vi "test_CONEX.vi"() -> ()   [LabVIEW 2010]
uses:
  <vilib>/Utility/inputDevices.llb/mouseAcquire.vi
  <vilib>/Utility/inputDevices.llb/closeMouse.vi
panel:
  in  "stop moving":bool
  in  "mouse sensitivity":dbl(slide)=4.94949494949495 scale=0.0..10.0
  in  "move with mouse":bool
  in  "Units":enum16{"mm", "um", "nm"}(ring)=enum."um"
  in  "Goto (incr)":bool
  in  "Motors to move":bool[](array[boolean])=[TRUE, TRUE, TRUE]
  in  "Incr. Stage Move (um)":dbl[](array[numeric])=[0.0, 0.0, 0.0]
  out "moving stage?":bool
  in  "Retract Limit":dbl[](array[numeric])=[0.0, 0.0, 0.0]
  in  "Extend Limit":dbl[](array[numeric])=[12.0, 12.0, 12.0]
  out "Position (mm)":dbl[](array[numeric]) format="%.5g"
  out "CONEX Cluster":T1
  in  "Connected devices":string[](array[string])=["COM3", "COM4", "COM5"]
  in  "Controller Addresses":i32[](array[numeric])=[1, 1, 1]
  in  "Abs. Stage Move":dbl[](array[numeric])=[0.0, 0.0, 0.0]
  in  "Goto (abs)":bool
  in  "stop":bool
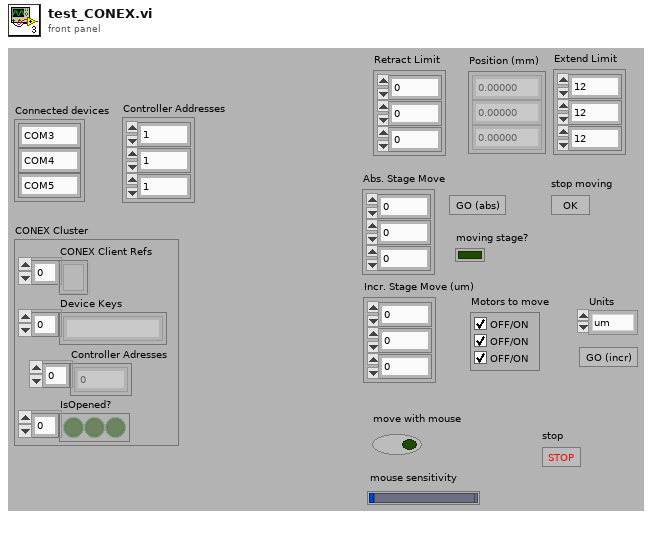
[diagram p1: front panel]
types:
  T1 = cluster{"CONEX Client Refs":refnum<k24>[], "Device Keys":string[], "Controller Adresses":i32[], "IsOpened?":bool[]}
  T2 = cluster{"Horizontal":i32, "Vertical":i32, "Scrolling":i32}
  T3 = cluster{"button 1":bool, "button 2":bool, "button 3":bool, "button 4":bool}
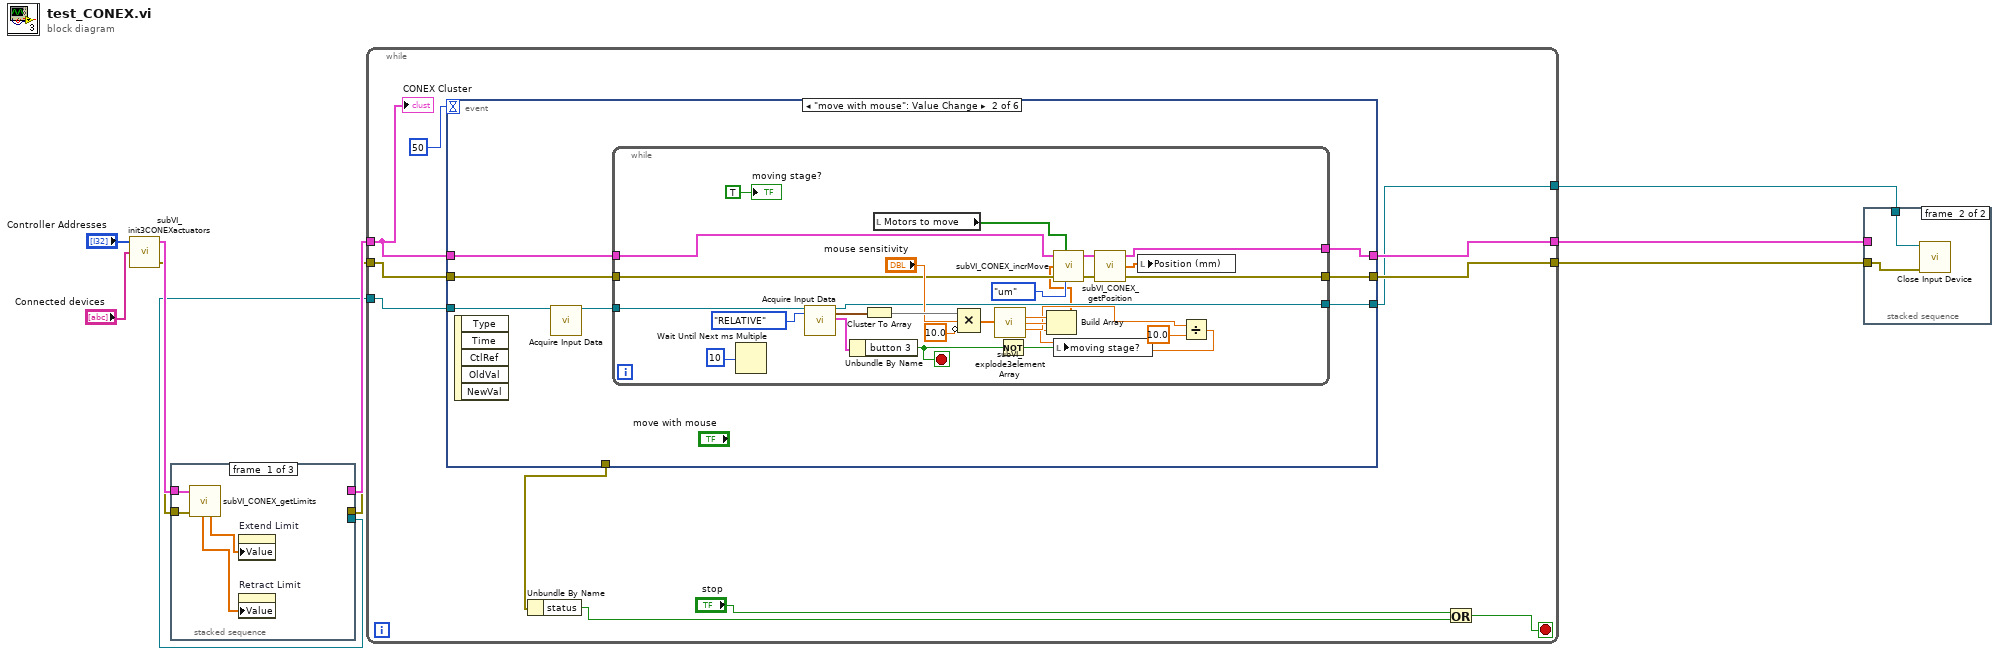
[diagram p0: block diagram]
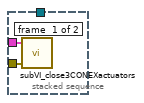
[diagram p2: hidden frame]
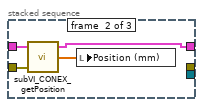
[diagram p3: hidden frame]
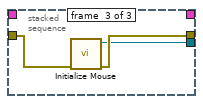
[diagram p4: hidden frame]
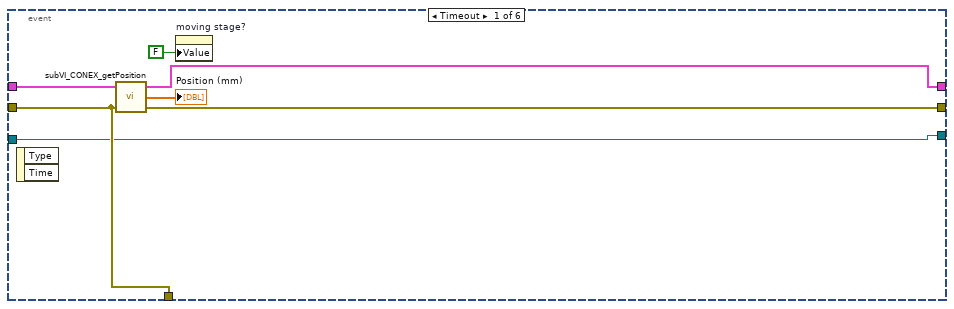
[diagram p5: hidden frame]
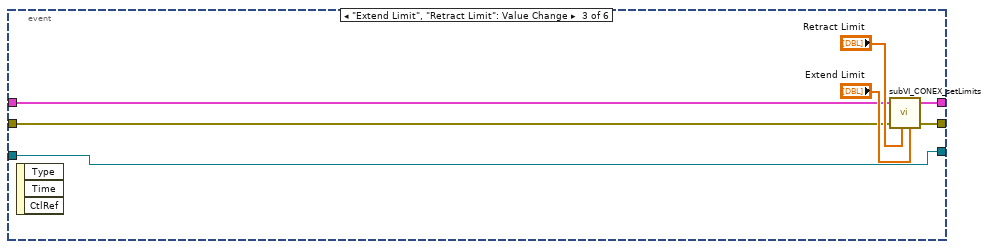
[diagram p6: hidden frame]
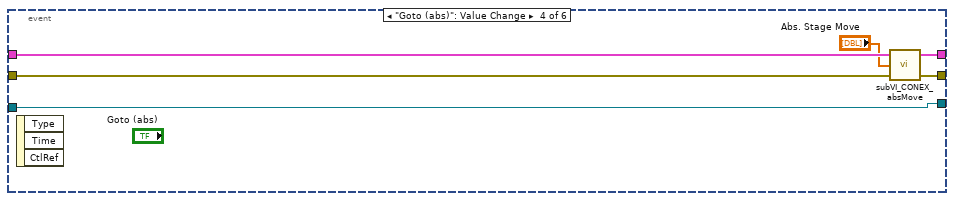
[diagram p7: hidden frame]
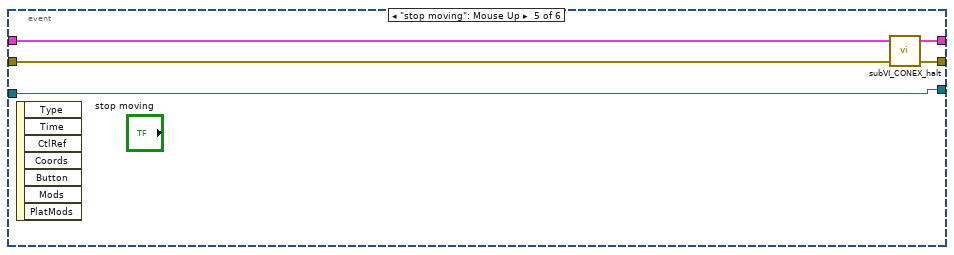
[diagram p8: hidden frame]
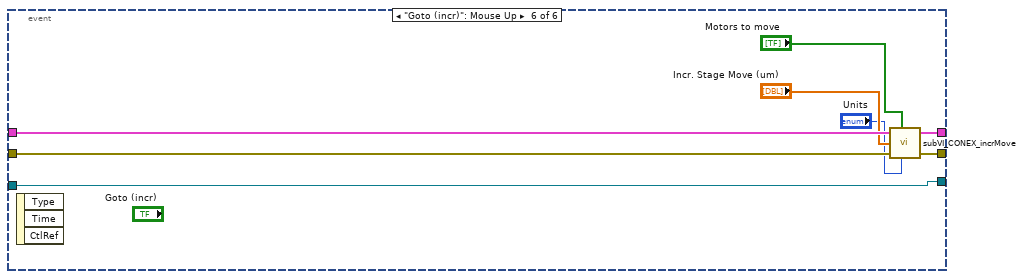
[diagram p9: hidden frame]
diagram:
  n1 = call "subVI_init3CONEXactuators.vi"("Connected devices"="Connected devices", "Controller Addresses"="Controller Addresses") -> ("Error OUT"=w6:errorcluster, "CONEX Cluster"=w7:T1)  [unwired: 2 in]
  n2 = stacked-sequence {
    tunnel: w7 -> [w14 w17 _]
    tunnel: w6 -> [w13 w16 w21]
    tunnel: [_ w15 _] -> w5
    tunnel: [_ _ w20] -> w4
    tunnel: [_ _ w19] -> w2
    frame #0 {
      n3 = call "subVI_CONEX_getLimits.vi"("CONEX Cluster"=w14, "Error IN"=w13) -> ("Retract Limit"=w11:dbl[], "Extend Limit"=w12:dbl[])  [unwired: 4 in, 2 out]
      n4 = property on="Extend Limit" class="Arr (strict)"("Value"=w12) -> ()  [unwired: 2 in, 2 out]
      n5 = property on="Retract Limit" class="Arr (strict)"("Value"=w11) -> ()  [unwired: 2 in, 2 out]
    }
    frame #1 {
      n6 = call "subVI_CONEX_getPosition.vi"("Error IN"=w16, "CONEX Cluster"=w17) -> ("Current Position (mm)"=w18:dbl[], "CONEX Cluster out"=w15:T1)  [unwired: 1 in, 1 out]
      n7 = local write "Position (mm)"(w18) -> ()
    }
    frame #2 {
      n8 = call <vilib>:"Initialize Mouse.vi"("error in (no error)"=w21) -> ("error out"=w20:errorcluster, "device ID"=w19:refnum<k1>)  [unwired: 9 in]
    }
  }
  n9 = while {
    tunnel: w5 -> [w31]
    tunnel: w4 -> [w30]
    tunnel: [w29] -> w10
    tunnel: [w28] -> w3
    tunnel: w2 -> [w23]
    tunnel: [w22] -> w1
    stop <- w24 stop-if-true
    n10 = event shown="[1] \"move with mouse\": Value Change" {
      selector: _ -> [_ _ _ _ _ _]
      dyn-events: _ -> [_ _ _ _ _ _]
      timeout: 50 -> [_ _ _ _ _ _]
      tunnel: w31 -> [w39 w46 w79 w87 w92 w100]
      tunnel: w30 -> [w36 w45 w78 w86 w91 w99]
      tunnel: [w33 w43 w77 w85 w89 w97] -> w29
      tunnel: [w34 w44 w76 w84 w90 w98] -> w28
      tunnel: [w36 _ _ _ _ _] -> w27
      tunnel: w23 -> [w35 w41 w75 w83 w88 w93]
      tunnel: [w35 w42 w75 w83 w88 w93] -> w22
      event Timeout {
        n11 = event-data() -> ()  [unwired: 1 in, 2 out]
        n12 = call "subVI_CONEX_getPosition.vi"("Error IN"=w36, "CONEX Cluster"=w39) -> ("error out"=w33:errorcluster, "Current Position (mm)"=→"Position (mm)":dbl[], "CONEX Cluster out"=w34:T1)  [unwired: 1 in]
        n13 = property on="moving stage?" class="Bool (strict)"("Value"=FALSE ("Boolean")) -> ()  [unwired: 2 in, 2 out]
      }
      event "move with mouse": Value Change {
        n14 = event-data() -> ()  [unwired: 1 in, 5 out]
        n15 = call-poly <vilib>:"Acquire Input Data.vi"("device ID"=w41) -> ("device ID"=w40:refnum<k1>)  [unwired: 15 in, 3 out]
        n16 = while {
          tunnel: w46 -> [w65]
          tunnel: w45 -> [w66]
          tunnel: [w60] -> w44
          tunnel: [w59] -> w43
          tunnel: w40 -> [w74]
          tunnel: [w54] -> w42
          stop <- w55 stop-if-true
          n17 = Wait Until Next ms Multiple(millisecond multiple=u32 10) -> ()  [unwired: 1 out]
          n18 = call-poly <vilib>:"Acquire Input Data.vi"("device ID"=w74, "key mode"=enum16{"RELATIVE", "ABSOLUTE"}."RELATIVE") -> ("device ID"=w54:refnum<k1>, "axis info"=w71:T2, "button info"=w63:T3)  [unwired: 14 in, 1 out]
          n19 = Unbundle By Name(w63) -> ("button 3"=w55:bool)
          n20 = Cluster To Array(cluster=w71) -> (array=w70:i32[])
          n21 = local read "Motors to move"() -> (w64:bool[])
          n22 = Compound Arithmetic op=MULTIPLY(w70, "mouse sensitivity", invert 10.0 ("value")) -> (w53:dbl[])
          n23 = call "subVI_explode3elementArray.vi"("Array"=w53) -> ("x"=w52:dbl, "y"=w51:dbl, "z"=w49:dbl)  [unwired: 12 in]
          n24 = Not(x=w55) -> (.not. x?=w56:bool)
          n25 = local write "moving stage?"(w56) -> ()
          n26 = Divide(x=w49, y=10.0) -> (x/y=w48:dbl)
          n27 = Build Array(w52, w51, w48) -> (w47:dbl[])
          n28 = call "subVI_CONEX_incrMove.vi"("CONEX Cluster"=w65, "Motors to move"=w64, "Incr. Move (um default)"=w47, "Error IN"=w66, "Units"=enum16{"mm", "um", "nm"}."um") -> ("CONEX Cluster out"=w62:T1, "error out"=w61:errorcluster)  [unwired: 3 in]
          n29 = call "subVI_CONEX_getPosition.vi"("Error IN"=w61, "CONEX Cluster"=w62) -> ("error out"=w59:errorcluster, "Current Position (mm)"=w58:dbl[], "CONEX Cluster out"=w60:T1)  [unwired: 1 in]
          n30 = local write "Position (mm)"(w58) -> ()
          "moving stage?" <- TRUE ("moving stage?")
        }
      }
      event "Extend Limit", "Retract Limit": Value Change {
        n31 = event-data() -> ()  [unwired: 1 in, 3 out]
        n32 = call "subVI_CONEX_setLimits.vi"("CONEX Cluster"=w79, "Error IN"=w78, "Retract Limit"="Retract Limit", "Extend Limit"="Extend Limit") -> ("CONEX Cluster out"=w76:T1, "error out"=w77:errorcluster)  [unwired: 4 in]
      }
      event "Goto (abs)": Value Change {
        n33 = event-data() -> ()  [unwired: 1 in, 3 out]
        n34 = call "subVI_CONEX_absMove.vi"("Error IN"=w86, "Target Pos."="Abs. Stage Move", "CONEX Cluster"=w87) -> ("error out"=w85:errorcluster, "CONEX Cluster out"=w84:T1)  [unwired: 1 in]
      }
      event "stop moving": Mouse Up {
        n35 = event-data() -> ()  [unwired: 1 in, 7 out]
        n36 = call "subVI_CONEX_halt.vi"("Error IN"=w91, "CONEX Cluster"=w92) -> ("error out"=w89:errorcluster, "CONEX Cluster out"=w90:T1)  [unwired: 2 in]
      }
      event "Goto (incr)": Mouse Up {
        n37 = event-data() -> ()  [unwired: 1 in, 3 out]
        n38 = call "subVI_CONEX_incrMove.vi"("CONEX Cluster"=w100, "Motors to move"="Motors to move", "Incr. Move (um default)"="Incr. Stage Move (um)", "Error IN"=w99, "Units"="Units") -> ("CONEX Cluster out"=w98:T1, "error out"=w97:errorcluster)  [unwired: 3 in]
      }
    }
    n39 = Unbundle By Name(w27) -> ("status"=w25:bool)
    n40 = Or(x="stop", y=w25) -> (x .or. y?=w24:bool)
    "CONEX Cluster" <- w31
  }
  n41 = stacked-sequence {
    tunnel: w10 -> [w102 w103]
    tunnel: w3 -> [w101 _]
    tunnel: w1 -> [_ w104]
    frame #0 {
      n42 = call "subVI_close3CONEXactuators.vi"("error in (no error)"=w102, "CONEX Cluster"=w101) -> ()  [unwired: 3 in, 1 out]
    }
    frame #1 {
      n43 = call-poly <vilib>:"Close Input Device.vi"("error in (no error)"=w103, "device ID"=w104) -> ()  [unwired: 8 in, 1 out]
    }
  }
